vi "Find Turntable Centre.vi"(3 "Mode":T6=enum."Run VI", 5 "Traverse line In":T3={"Start X"=-1250.0, "Start Y"=-250.0, "Start Z"=180.0, "End X"=0.0, "End Y"=0.0, "End Z"=0.0, "No. of pts."=6, "Spacing"=enum."Linear", "Filename"=path "C:/Enflo_Data_Local/2015/EnFlo_Tunnel/Paul_Hayden/Calibrations/Cal_06-2015/Datum_Block_1.xls", "Tunnel Speed"=0.0, "Averaging time (min)"=0.01, "Extra Commands"="", "Carrier_1 Q (l/min)"=nan, "Carrier_2 Q (l/min)"=nan, "Trace Gas Concentration (%)"=nan, "Specific Arguments"="Datum_Image_Calibration.vi  ", "Comments"="", "Row No"=0, "Row Type Selector"=enum."Run VI Named:", "Completion time"="12:51  12-06-2015", "Row Duration (mins)"=0.11291999999999999, "No. of Valid pts."=6, "Meas Setup File"="Trav_Cam_Picture.xls"} {"Carrier_2 Q (l/min)" format="%#.2f"; "Row Duration (mins)" format="%#.1f"; "Row No" min=0; "Trace Gas Concentration (%)" min=0.0 format="%#_4f"; "Carrier_1 Q (l/min)" format="%#.2f"; "Tunnel Speed" format="%#.2f"; "Start X" format="%#.2f"; "Start Y" format="%#.2f"; "Start Z" format="%#.2f"; "End X" format="%#.2f"; "End Y" format="%#.2f"; "End Z" format="%#.2f"; "Averaging time (min)" min=0.0 format="%#.2f"}) -> (0 "Error Message":string, 1 "Status":T2, 2 "Traverse line Out":T3 {"Carrier_2 Q (l/min)" format="%#.2f"; "Row Duration (mins)" format="%#.1f"; "Row No" min=0; "Trace Gas Concentration (%)" min=0.0 format="%#_4f"; "Carrier_1 Q (l/min)" format="%#.2f"; "Tunnel Speed" format="%#.2f"; "Start X" format="%#.2f"; "Start Y" format="%#.2f"; "Start Z" format="%#.2f"; "End X" format="%#.2f"; "End Y" format="%#.2f"; "End Z" format="%#.2f"; "Averaging time (min)" min=0.0 format="%#.2f"})   [LabVIEW 2015]
uses:
  Gen Trav/Traverse_cluster.ctl
  Gen Trav/Spacing.ctl
  Controls/Multi_run_mode.ctl
  Controls/User_Specific_mode.ctl
  Gen Trav/Multi_Run_Status.ctl
  Camera Server/Camera enum/Camera enum.ctl
  Utilities/Image acquisition and processing/Feature detection/Typedefs/Top level controls.ctl
  Utilities/Image acquisition and processing/Feature detection/Typedefs/Theta range.ctl
  Utilities/Image acquisition and processing/Feature detection/Typedefs/Txy range.ctl
  Utilities/Image acquisition and processing/Feature detection/Typedefs/ROI bounds.ctl
  Controls/Setup.ctl
  Controls/Save_Data.ctl
  Globals/Trav_pos_global.vi
  Globals/Constants_global.vi
  Globals/Dynamic_call_global.ph.vi
panel:
  in  "Camera":T1="Travcam"
  out "Local Log File":path
  out "y radius":dbl
  out "x radius":dbl
  out "y centre 2":dbl
  out "x centre 2":dbl
  in  "stop":bool
  out "radius":dbl
  out "y centre":dbl
  out "x centre":dbl
  out "Y":dbl[](array[numeric])
  out "X":dbl[](array[numeric])
  in  "X Offset from Camera":dbl=50.0
  in  "Radius":dbl=500.0
  # "Circle"
  # "Ellipse"
  # "X           Y            Z"
  # "Start"
  # "End"
  # "X           Y            Z"
  # "Start"
  # "End"
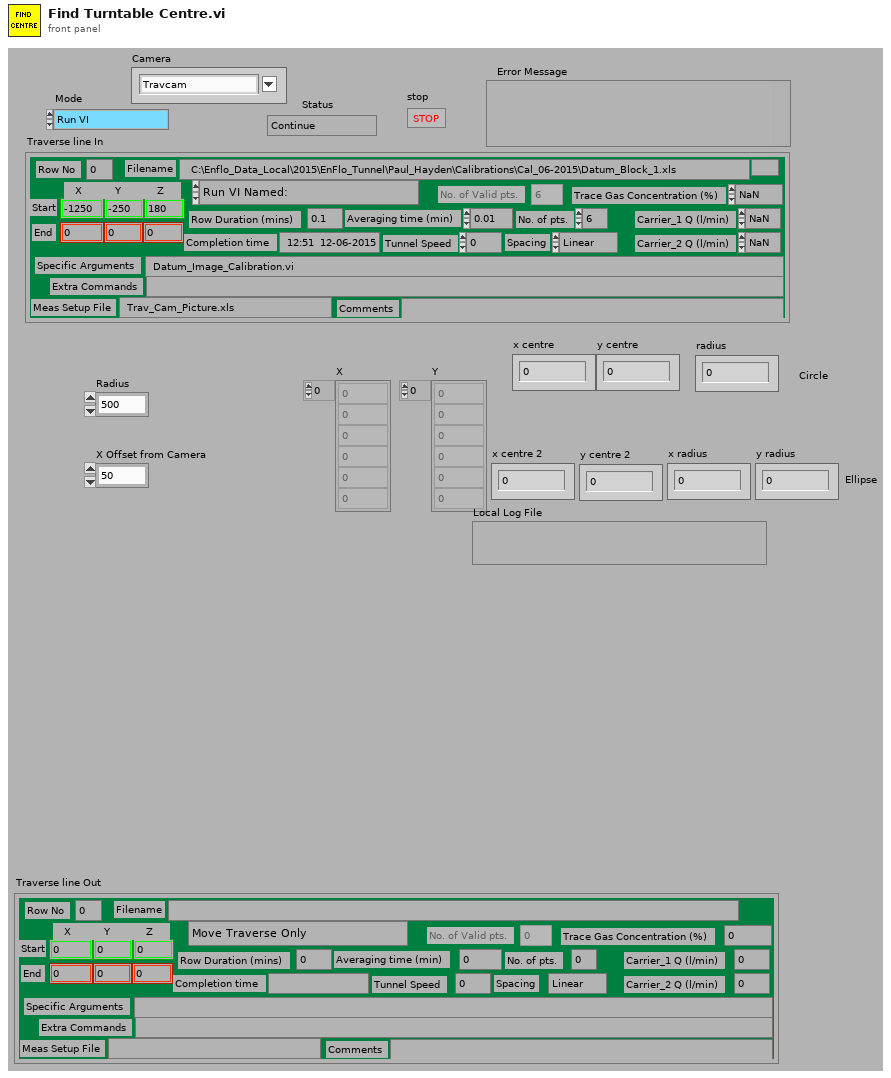
[diagram p1: front panel]
types:
  T1 = typedef "Camera enum.ctl" = string
  T2 = typedef "Multi_Run_Status.ctl" = enum16{"Continue", "Jump to Next Point", "Jump to Next Row", "Jump To Fall Back", "Terminate Run"}
  T3 = typedef "Traverse_cluster.ctl" = cluster{"Start X":sgl, "Start Y":sgl, "Start Z":sgl, "End X":sgl, "End Y":sgl, "End Z":sgl, "No. of pts.":i32, "Spacing":T4, "Filename":path, "Tunnel Speed":dbl, "Averaging time (min)":dbl, "Extra Commands":string, "Carrier_1 Q (l/min)":dbl, "Carrier_2 Q (l/min)":dbl, "Trace Gas Concentration (%)":dbl, "Specific Arguments":string, "Comments":string, "Row No":i32, "Row Type Selector":T5, "Completion time":string, "Row Duration (mins)":dbl, "No. of Valid pts.":i32, "Meas Setup File":string}
  T4 = typedef "Spacing.ctl" = enum16{"Linear", "Log", "Gauss", "Specified", "N/A"}
  T5 = typedef "Multi_run_mode.ctl" = enum16{"Move Traverse Only", "Set Tunnel Speed Only", "Set Source Only", "Set Measurement Conditions", "Single Measurement", "Vertical Profile", "Lateral Profile", "Longitudinal Profile", "Explore Volume", "Multi-Axis Profile", "Auto Calibrate", "Meas Fast FID Bkgnd", "Check Beam Power", "Scanning Valve Measurement", "Run VI Named:", "Set ADAM Ch", "Wait (minutes)", "Send Message", "Synchronize With:", "Fall Back to this Row", "Turn Off Row Repeating", "Blank Row", "Traverse 3D Volume"}
  T6 = typedef "User_Specific_mode.ctl" = enum16{"Check VI only", "Run VI"}
  T7 = typedef "ROI bounds.ctl" = cluster{"Xmax":i32, "Ymax":i32, "Xmin":i32, "Ymin":i32}
  T8 = typedef "Txy range.ctl" = cluster{"Tx max (pix)":i32, "Tx min (pix)":i32, "Ty max (pix)":i32, "Ty min (pix)":i32}
  T9 = typedef "Theta range.ctl" = cluster{"theta max (deg)":dbl, "theta min (deg)":dbl}
  T10 = typedef "Top level controls.ctl" = cluster{"Auto ROI (for rot.)":bool, "Apply scaling":bool, "Apply rotation":bool, "Apply Tx":bool, "Apply Ty":bool, "Keep proc. img":bool}
  T11 = typedef "Save_Data.ctl" = enum16{"Save No Data", "Save Data"}
  T12 = typedef "Setup.ctl" = enum16{"Run Program", "Show Setup", "Save Current Setup", "Setup Front Panel"}
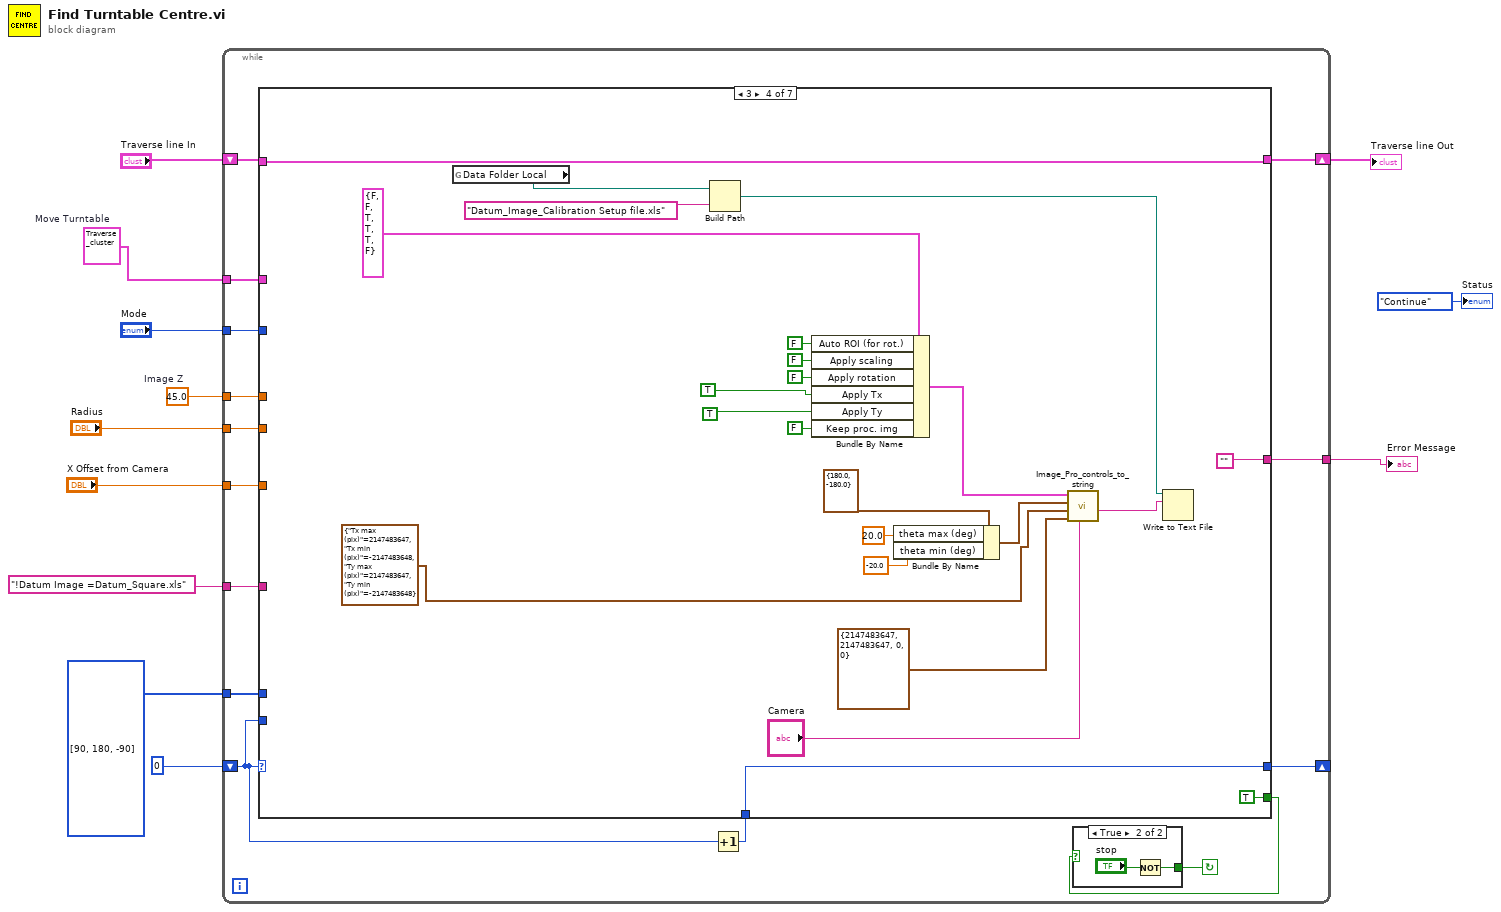
[diagram p0: block diagram]
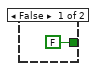
[diagram p2: hidden frame]
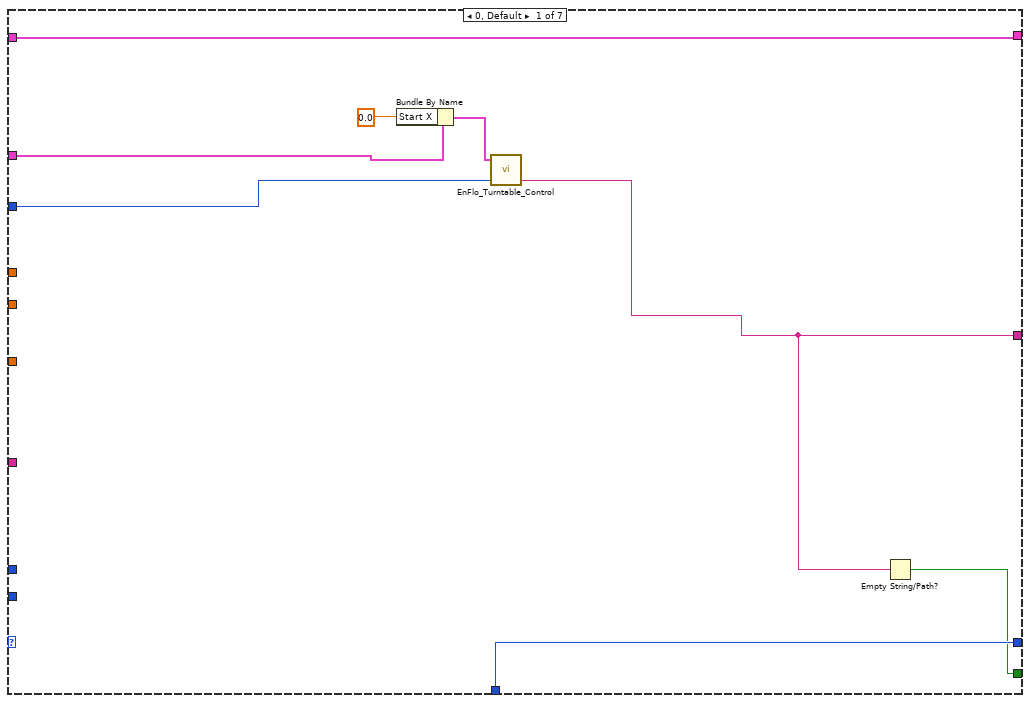
[diagram p3: hidden frame]
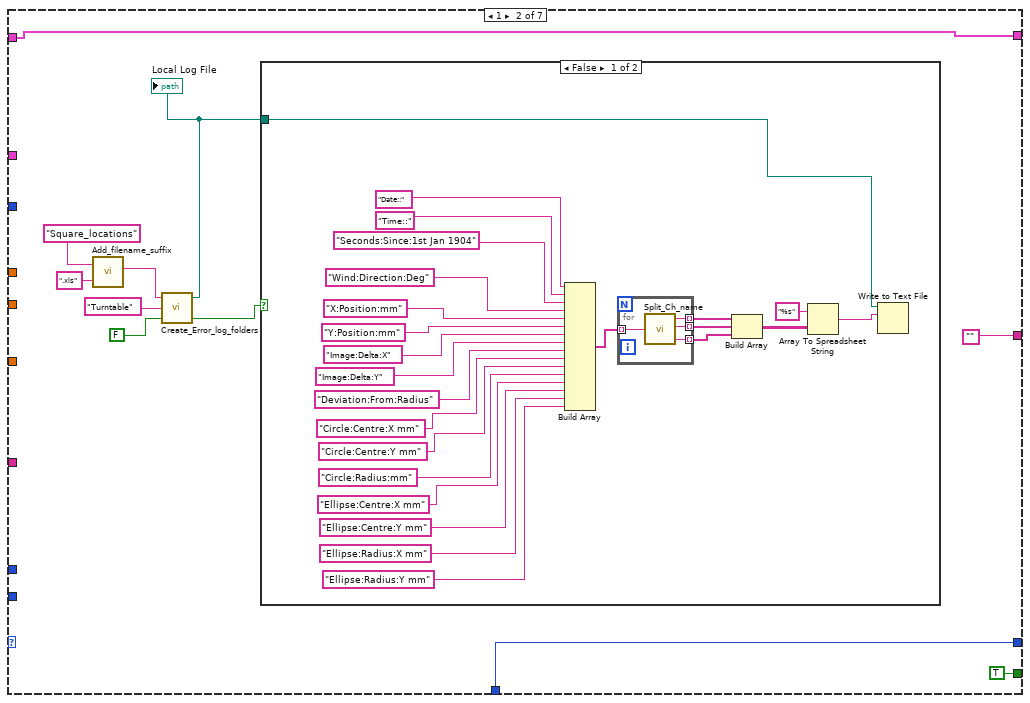
[diagram p4: hidden frame]
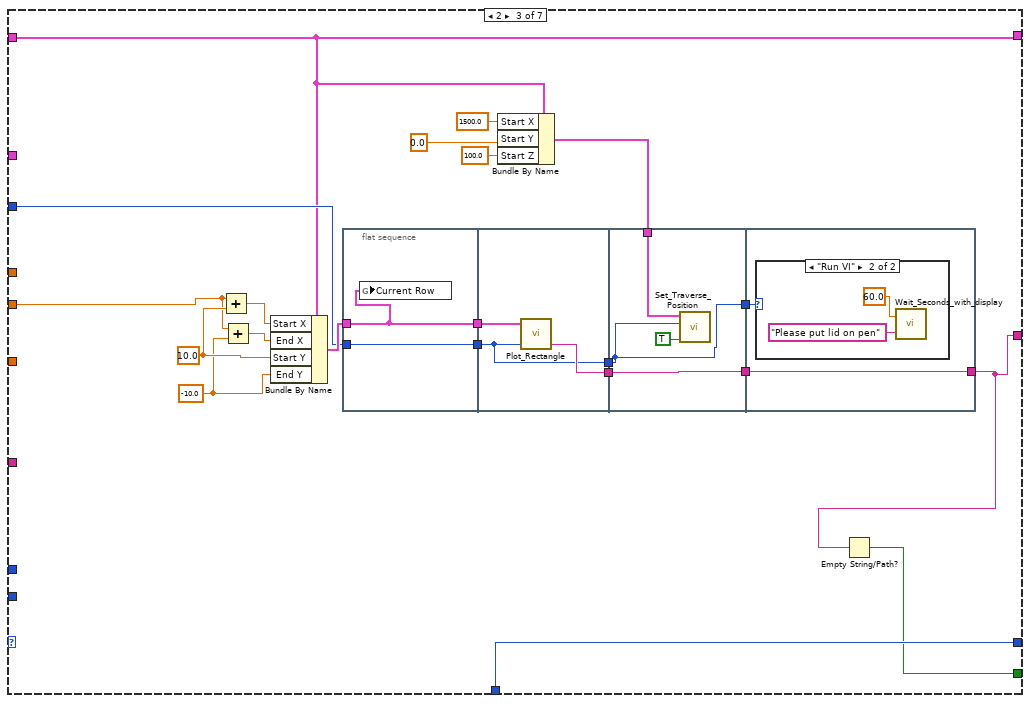
[diagram p6: hidden frame]
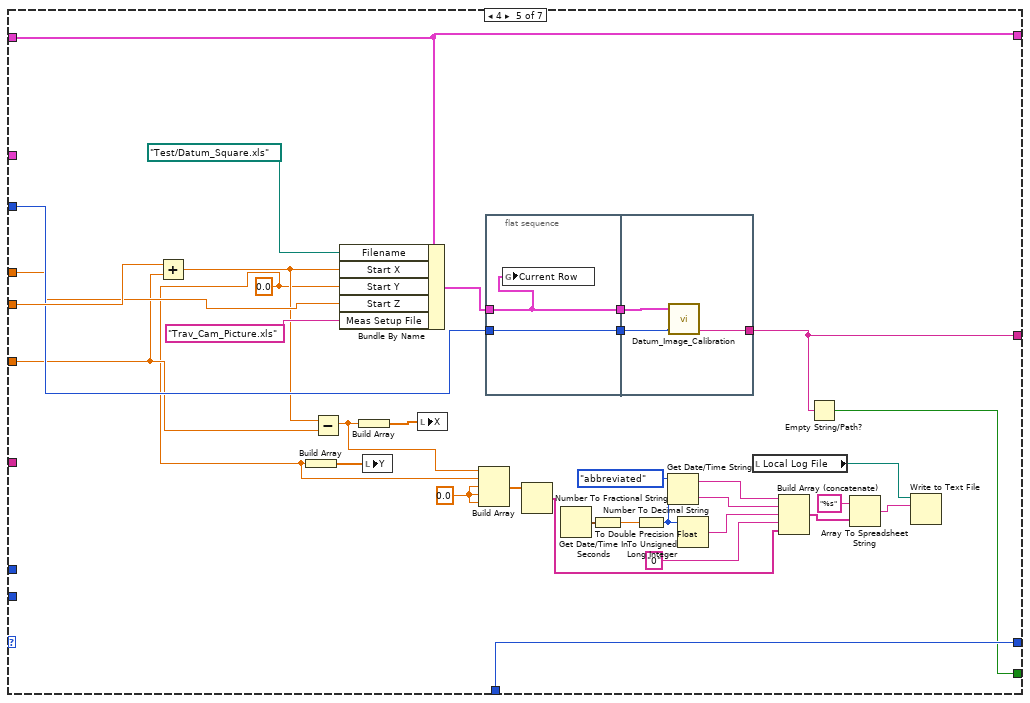
[diagram p8: hidden frame]
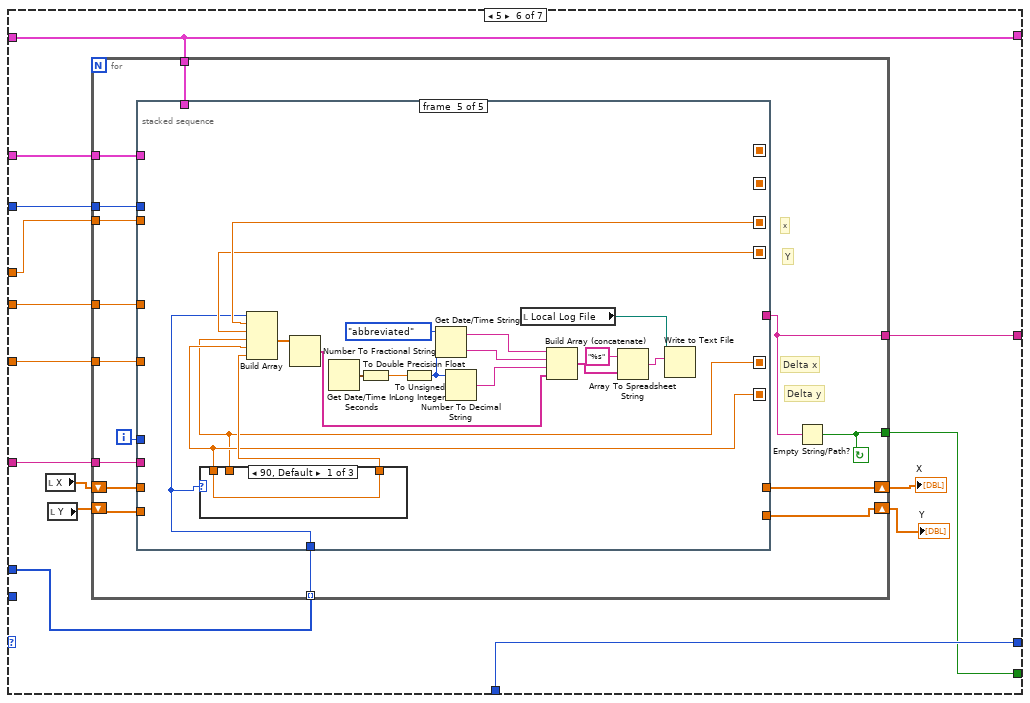
[diagram p9: hidden frame]
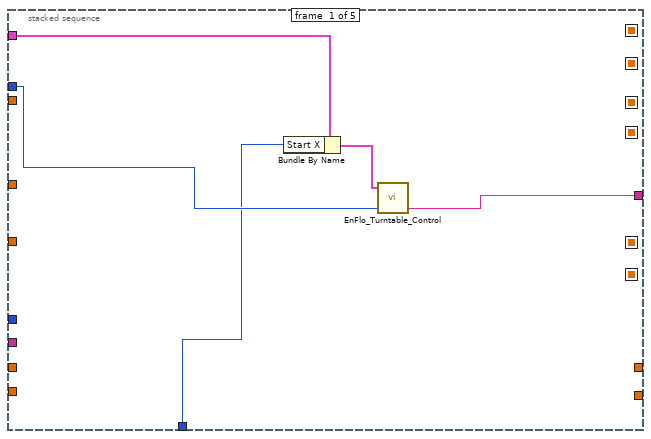
[diagram p10: hidden frame]
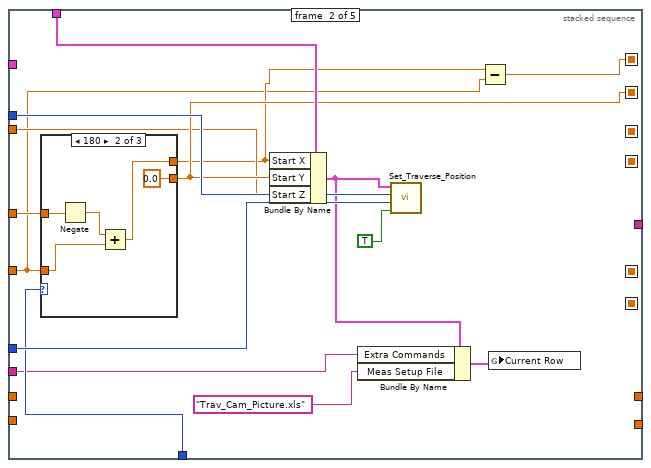
[diagram p11: hidden frame]
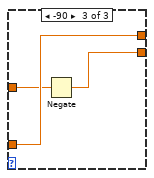
[diagram p13: hidden frame]
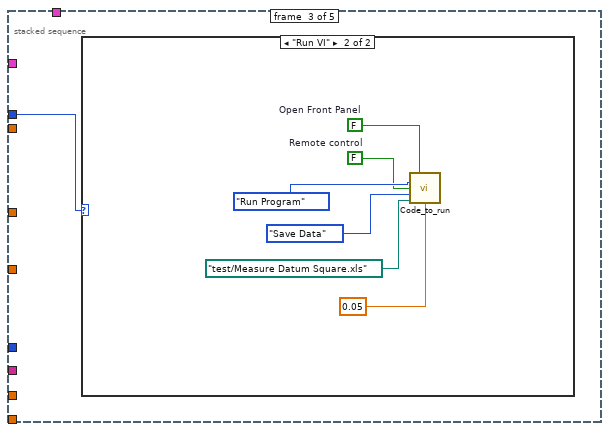
[diagram p14: hidden frame]
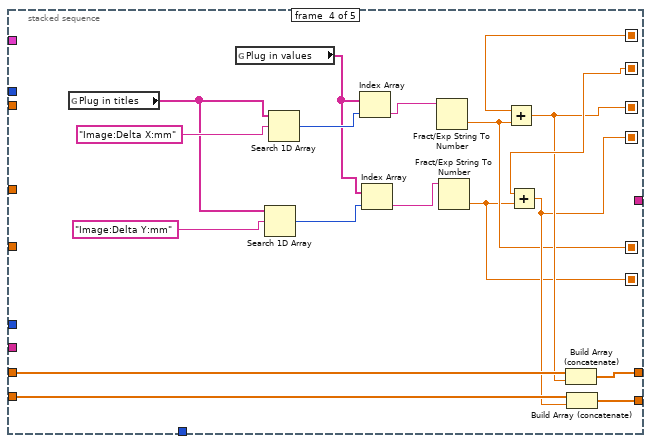
[diagram p16: hidden frame]
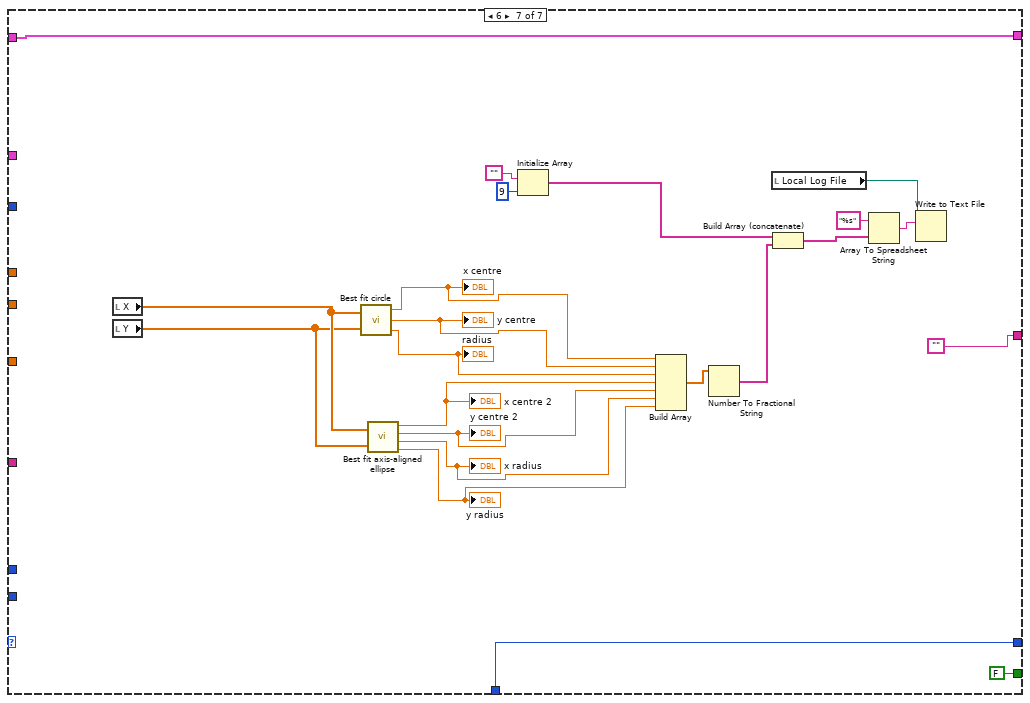
[diagram p19: hidden frame]
diagram:
  w1 = T3 {"Start X"=0.0, "Start Y"=nan, "Start Z"=nan, "End X"=nan, "End Y"=nan, "End Z"=nan, "No. of pts."=0, "Spacing"=enum."N/A", "Filename"=path "  ---------", "Tunnel Speed"=nan, "Averaging time (min)"=nan, "Extra Commands"="!Datum Image = Datum_Turntable.xls", "Carrier_1 Q (l/min)"=nan, "Carrier_2 Q (l/min)"=nan, "Trace Gas Concentration (%)"=nan, "Specific Arguments"="EnFlo_Turntable_Control.vi", "Comments"="", "Row No"=0, "Row Type Selector"=enum."Run VI Named:", "Completion time"="18:36  07-04-2016", "Row Duration (mins)"=0.6666666666666666, "No. of Valid pts."=0, "Meas Setup File"="Trav_Cam_Picture.xls"}  # Move Turntable
  w4 = sgl 45.0  # Image Z
  n1 = while {
    shift-left: 0 -> [w23]
    shift-right: [w27] -> _
    tunnel: "Mode" -> [w26]
    shift-right: [w24] -> w9
    shift-left: "Traverse line In" -> [w25]
    tunnel: "Radius" -> [w21]
    tunnel: "X Offset from Camera" -> [w20]
    tunnel: [w19] -> w6
    tunnel: w4 -> [w18]
    tunnel: i32[] [90, 180, -90] ("appended array") -> [w15]
    tunnel: "!Datum Image =Datum_Square.xls" ("Extra Commands") -> [w14]
    tunnel: w1 -> [w13]
    stop <- w16 continue-if-true
    n2 = Increment(x=w23) -> (x+1=w22:i32)
    n3 = case shown="3" w23 {
      tunnel: [w36 TRUE w95 TRUE w162 w184 FALSE] -> w17
      tunnel: [w38 w41 w97 w134 w166 w187 w298] -> w27
      tunnel: w23 -> [_ _ _ _ _ _ _]
      tunnel: w26 -> [w35 _ w96 _ w158 w186 _]
      tunnel: w25 -> [w37 w42 w86 w133 w167 w181 w299]
      tunnel: [w37 w42 w86 w133 w167 w181 w299] -> w24
      tunnel: w22 -> [w38 w41 w97 w134 w166 w187 w298]
      tunnel: w21 -> [_ _ w89 _ w164 w182 _]
      tunnel: w20 -> [_ _ _ _ w144 w183 _]
      tunnel: [w32 "" w79 "" w157 w185 ""] -> w19
      tunnel: w18 -> [_ _ _ _ w154 w176 _]
      tunnel: w15 -> [_ _ _ _ _ w175 _]
      tunnel: w14 -> [_ _ _ _ _ w174 _]
      tunnel: w13 -> [w31 _ _ _ _ w173 _]
      frame 0, Default {
        n4 = Bundle By Name(cluster=w31, "Start X"=sgl 0.0 ("element")) -> (w34:T3)
        n5 = call "EnFlo_Turntable_Control.vi"("Mode"=w35, "Traverse line In"=w34) -> ("Error Message"=w32:string)  [unwired: 1 in, 2 out]
        n6 = Empty String/Path?(string/path=w32) -> (empty?=w36:bool)
      }
      frame 1 {
        n7 = call "Add_filename_suffix.vi"("Filename"="Square_locations", "Suffix to add"=".xls") -> ("Filename out"=w47:string)  [unwired: 3 out]
        n8 = call "Create_Error_log_folders.vi"("Per Day Log File?"=FALSE, "Log Folder"="Turntable" ("Input Element"), "Log Filename"=w47) -> ("exists?"=w45:bool, "Local Log File"=w43:path)  [unwired: 1 out]
        "Local Log File" <- w43
        n9 = case shown="False" w45 {
          tunnel: w43 -> [w60 _]
          frame False {
            n10 = Build Array("Date::", "Time::", "Seconds:Since:1st Jan 1904", "Wind:Direction:Deg", "X:Position:mm", "Y:Position:mm", "Image:Delta:X", "Image:Delta:Y", "Deviation:From:Radius", "Circle:Centre:X mm", "Circle:Centre:Y mm", "Circle:Radius:mm", "Ellipse:Centre:X mm", "Ellipse:Centre:Y mm", "Ellipse:Radius:X mm", "Ellipse:Radius:Y mm") -> (w69:string[])
            n11 = for {
              tunnel: w69 -> [w77] mode=indexing
              tunnel: [w76] -> w68 mode=indexing
              tunnel: [w75] -> w67 mode=indexing
              tunnel: [w74] -> w66 mode=indexing
              n12 = call "Split_Ch_name.vi"("Ch name"=w77) -> ("Top level"=w76:string, "Middle"=w75:string, "Low level"=w74:string)
            }
            n13 = Build Array(w68, w67, w66) -> (w58:string[][])
            n14 = Array To Spreadsheet String(array=w58, 3:"%s" ("format string")) -> (spreadsheet string=w57:string)  [unwired: 1 out]
            n15 = Write to Text File(file (use dialog)=w60, text=w57) -> ()  [unwired: 2 in, 3 out]
          }
          frame True {
          }
        }
      }
      frame 2 {
        w90 = sgl -10.0 ("End Y")
        w91 = sgl 10.0 ("Start Y")
        n16 = Add(x=w89, y=w91) -> (x+y=w92:dbl)
        n17 = Add(x=w89, y=w90) -> (x+y=w88:dbl)
        n18 = Bundle By Name(cluster=w86, "Start X"=w92, "End X"=w88, "Start Y"=w91, "End Y"=w90) -> (w98:T3)
        n19 = flat-sequence {
          tunnel: w96 -> [w100]
          tunnel: w98 -> [w99]
          tunnel: [w99] -> w94
          tunnel: [w100] -> w93
          tunnel: w94 -> [w103]
          tunnel: w93 -> [w101]
          tunnel: [w102] -> w87
          tunnel: [w101] -> w81
          tunnel: w87 -> [w107]
          tunnel: w82 -> [w106]
          tunnel: w81 -> [w104]
          tunnel: [w107] -> w80
          tunnel: [w104] -> w78
          tunnel: [w109] -> w79
          tunnel: w80 -> [w109]
          tunnel: w78 -> [w108]
          frame #0 {
            n20 = global write "Trav_pos_global.vi" "Current Row"(w99) -> ()
          }
          frame #1 {
            n21 = call "Plot_Rectangle.vi"("Mode"=w101, "Traverse line In"=w103) -> ("Error Message"=w102:string)  [unwired: 1 in, 2 out]
          }
          frame #2 {
            n22 = call "Set_Traverse_Position.vi"("Last Part of Move?"=TRUE, "Simulate/Run"=w104, "Traverse line"=w106) -> ()  [unwired: 3 in, 1 out]
          }
          frame #3 {
            n23 = case shown="\"Run VI\"" w108 {
              frame "Check VI only" {
              }
              frame "Run VI" {
                n24 = call "Wait_Seconds_with_display.vi"("Message"="Please put lid on pen", "Seconds to wait"=60.0) -> ()  [unwired: 1 in, 1 out]
              }
            }
          }
        }
        n25 = Bundle By Name(cluster=w86, "Start X"=sgl 1500.0, "Start Y"=sgl 0.0, "Start Z"=sgl 100.0) -> (w82:T3)
        n26 = Empty String/Path?(string/path=w79) -> (empty?=w95:bool)
      }
      frame 3 {
        n27 = global read "Constants_global.vi" "Data Folder Local"() -> (w131:path)
        n28 = Build Path(base path=w131, name or relative path="Datum_Image_Calibration Setup file.xls") -> (appended path=w115:path)
        n29 = Bundle By Name(cluster=T10 {"Auto ROI (for rot.)"=FALSE, "Apply scaling"=FALSE, "Apply rotation"=TRUE, "Apply Tx"=TRUE, "Apply Ty"=TRUE, "Keep proc. img"=FALSE} ("Controls"), "Auto ROI (for rot.)"=FALSE, "Apply scaling"=FALSE, "Apply rotation"=FALSE, "Apply Tx"=TRUE, "Apply Ty"=TRUE, "Keep proc. img"=FALSE) -> (w123:T10)
        n30 = Bundle By Name(cluster=T9 {"theta max (deg)"=180.0, "theta min (deg)"=-180.0} ("Theta range (deg)"), "theta max (deg)"=20.0, "theta min (deg)"=-20.0) -> (w121:T9)
        n31 = call "Image_Pro_controls_to_string.vi"("Camera"="Camera", "ROI to crop (pixels)"=T7 {"Xmax"=2147483647, "Ymax"=2147483647, "Xmin"=0, "Ymin"=0}, "Txy range (pixels)"=T8 {"Tx max (pix)"=2147483647, "Tx min (pix)"=-2147483648, "Ty max (pix)"=2147483647, "Ty min (pix)"=-2147483648}, "Theta range (deg)"=w121, "Controls"=w123) -> ("Setup String"=w116:string)  [unwired: 6 in]
        n32 = Write to Text File(file (use dialog)=w115, text=w116) -> ()  [unwired: 2 in, 3 out]
      }
      frame 4 {
        w141 = 0.0 ("element")
        w142 = sgl 0.0 ("Start Y")
        n33 = Add(x=w164, y=w144) -> (x+y=w145:dbl)
        n34 = Build Array(w142) -> (w155:sgl[])
        n35 = Subtract(x=w145, y=w144) -> (x-y=w143:dbl)
        n36 = Bundle By Name(cluster=w167, "Filename"=path "Test/Datum_Square.xls", "Start X"=w145, "Start Y"=w142, "Start Z"=w154, "Meas Setup File"="Trav_Cam_Picture.xls") -> (w159:T3)
        n37 = Build Array(w143) -> (w156:dbl[])
        n38 = local write "Y"(w155) -> ()
        n39 = local write "X"(w156) -> ()
        n40 = Build Array(w143, w142, w141, w141, w141) -> (w140:dbl[])
        n41 = flat-sequence {
          tunnel: w158 -> [w169]
          tunnel: w159 -> [w168]
          tunnel: [w168] -> w161
          tunnel: [w169] -> w160
          tunnel: [w170] -> w157
          tunnel: w161 -> [w172]
          tunnel: w160 -> [w171]
          frame #0 {
            n42 = global write "Trav_pos_global.vi" "Current Row"(w168) -> ()
          }
          frame #1 {
            n43 = call "Datum_Image_Calibration.vi"("Mode"=w171, "Traverse line In"=w172) -> ("Error Message"=w170:string)  [unwired: 1 in, 2 out]
          }
        }
        n44 = Number To Fractional String(number=w140) -> (F-format string=w139:string[])  [unwired: 3 in]
        n45 = Get Date/Time In Seconds() -> (seconds since 1Jan1904=w150:timestamp)
        n46 = To Double Precision Float(number=w150) -> (double precision float=w152:dbl)
        n47 = To Unsigned Long Integer(number=w152) -> (unsigned 32bit integer=w151:u32)
        n48 = Get Date/Time String(date format (0)=enum16{"short", "long", "abbreviated"}."abbreviated", seconds (now)=w151) -> (date string=w149:string, time string=w148:string)  [unwired: 1 out]
        n49 = Number To Decimal String(number=w151) -> (decimal integer string=w147:string)  [unwired: 1 out]
        n50 = local read "Local Log File"() -> (w138:path)
        n51 = Build Array (concatenate)(w149, w148, w147, "0", w139) -> (w136:string[])
        n52 = Empty String/Path?(string/path=w157) -> (empty?=w162:bool)
        n53 = Array To Spreadsheet String(array=w136, 3:"%s" ("format string")) -> (spreadsheet string=w135:string)  [unwired: 1 out]
        n54 = Write to Text File(file (use dialog)=w138, text=w135) -> ()  [unwired: 2 in, 3 out]
      }
      frame 5 {
        n55 = local read "X"() -> (w180:dbl[])
        n56 = local read "Y"() -> (w179:dbl[])
        n57 = for {
          tunnel: w186 -> [w202]
          tunnel: [w201] -> w185
          tunnel: [w200] -> w184
          tunnel: w175 -> [w199] mode=indexing
          tunnel: w183 -> [w198]
          tunnel: w182 -> [w197]
          tunnel: w181 -> [w196]
          shift-right: [w192] -> w178
          shift-left: w180 -> [w194]
          shift-right: [w191] -> w177
          shift-left: w179 -> [w193]
          tunnel: w176 -> [w190]
          tunnel: w174 -> [w189]
          tunnel: w173 -> [w188]
          i -> [w195]
          stop <- w200 continue-if-true
          # "Delta y"
          # "Delta x"
          # "Y"
          # "x"
          n58 = stacked-sequence {
            seq-local: [_ w211 _ _ _] -> [_ _ _ w249 _]
            seq-local: [_ w217 _ _ _] -> [_ _ _ w248 _]
            seq-local: [_ _ _ w243 _] -> [_ _ _ _ w263]
            seq-local: [_ _ _ w242 _] -> [_ _ _ _ w262]
            seq-local: [_ _ _ w241 _] -> [_ _ _ _ w258]
            seq-local: [_ _ _ w240 _] -> [_ _ _ _ w259]
            tunnel: w202 -> [w206 w221 w233 _ _]
            tunnel: [w203 _ _ _ _] -> w201
            tunnel: w199 -> [w205 w209 _ _ w261]
            tunnel: w198 -> [_ w210 _ _ _]
            tunnel: w197 -> [_ w218 _ _ _]
            tunnel: w196 -> [_ w222 _ _ _]
            tunnel: w195 -> [_ w219 _ _ _]
            tunnel: w194 -> [_ _ _ w247 _]
            tunnel: w193 -> [_ _ _ w246 _]
            tunnel: [_ _ _ w245 _] -> w192
            tunnel: [_ _ _ w244 _] -> w191
            tunnel: w190 -> [_ w213 _ _ _]
            tunnel: w189 -> [_ w208 _ _ _]
            tunnel: w188 -> [w204 _ _ _ _]
            frame #0 {
              n59 = Bundle By Name(cluster=w204, "Start X"=w205) -> (w207:T3)
              n60 = call "EnFlo_Turntable_Control.vi"("Mode"=w206, "Traverse line In"=w207) -> ("Error Message"=w203:string)  [unwired: 1 in, 2 out]
            }
            frame #1 {
              n61 = case shown="180" w209 {
                tunnel: w210 -> [w224 w226 w232]
                tunnel: [w224 w225 w232] -> w212
                tunnel: w218 -> [w223 w228 w231]
                tunnel: [w223 0.0 ("X position") w230] -> w217
                frame 90, Default {
                }
                frame 180 {
                  n62 = Negate(x=w228) -> (-x=w227:dbl)
                  n63 = Add(x=w227, y=w226) -> (x+y=w225:dbl)
                }
                frame -90 {
                  n64 = Negate(x=w231) -> (-x=w230:dbl)
                }
              }
              n65 = Bundle By Name(cluster=w222, "Start X"=w212, "Start Y"=w217, "Start Z"=w213) -> (w216:T3)
              n66 = Bundle By Name(cluster=w216, "Extra Commands"=w208, "Meas Setup File"="Trav_Cam_Picture.xls" ("Extra Commands")) -> (w215:T3)
              n67 = call "Set_Traverse_Position.vi"("Last Part of Move?"=TRUE, "Currently on Point"=w219, "Simulate/Run"=w221, "Traverse line"=w216) -> ()  [unwired: 2 in, 1 out]
              n68 = Subtract(x=w212, y=w210) -> (x-y=w211:dbl)
              n69 = global write "Trav_pos_global.vi" "Current Row"(w215) -> ()
            }
            frame #2 {
              n70 = case shown="\"Run VI\"" w233 {
                frame "Check VI only" {
                }
                frame "Run VI" {
                  w237 = FALSE  # Open Front Panel
                  w236 = FALSE  # Remote control
                  n71 = call "Code_to_run.vi"("Open Front Panel"=w237, "setup"=Setup."Run Program", "Remote control"=w236, "File"=Save_Data."Save Data", "Results Filename"=path "test/Measure Datum Square.xls", "Averaging time (min)"=0.05) -> ()  [unwired: 5 in, 5 out]
                }
              }
            }
            frame #3 {
              n72 = global read "Dynamic_call_global.ph.vi" "Plug in titles"() -> (w253:string[])
              n73 = global read "Dynamic_call_global.ph.vi" "Plug in values"() -> (w252:string[])
              n74 = Search 1D Array(1D array=w253, element="Image:Delta Y:mm") -> (index of element=w251:i32)  [unwired: 1 in]
              n75 = Search 1D Array(1D array=w253, element="Image:Delta X:mm") -> (index of element=w256:i32)  [unwired: 1 in]
              n76 = Index Array(array=w252, index=w256) -> (element=w257:string)
              n77 = Index Array(array=w252, index=w251) -> (element=w250:string)
              n78 = Fract/Exp String To Number(string=w257) -> (number=w241:dbl)  [unwired: 3 in, 1 out]
              n79 = Fract/Exp String To Number(string=w250) -> (number=w240:dbl)  [unwired: 3 in, 1 out]
              n80 = Add(x=w249, y=w241) -> (x+y=w243:dbl)
              n81 = Add(x=w248, y=w240) -> (x+y=w242:dbl)
              n82 = Build Array (concatenate)(w247, w243) -> (w245:dbl[])
              n83 = Build Array (concatenate)(w246, w242) -> (w244:dbl[])
            }
            frame #4 {
              n84 = case shown="90, Default" w261 {
                tunnel: [w277 w278 w279] -> w260
                tunnel: w259 -> [w277 w278 _]
                tunnel: w258 -> [_ _ w279]
                frame 90, Default {
                }
                frame -90 {
                }
                frame 180 {
                }
              }
              n85 = Build Array(w261, w263, w262, w258, w259, w260) -> (w269:dbl[])
              n86 = Number To Fractional String(number=w269) -> (F-format string=w268:string[])  [unwired: 3 in]
              n87 = Get Date/Time In Seconds() -> (seconds since 1Jan1904=w273:timestamp)
              n88 = To Double Precision Float(number=w273) -> (double precision float=w275:dbl)
              n89 = To Unsigned Long Integer(number=w275) -> (unsigned 32bit integer=w274:u32)
              n90 = Get Date/Time String(date format (0)=enum16{"short", "long", "abbreviated"}."abbreviated", seconds (now)=w274) -> (date string=w272:string, time string=w271:string)  [unwired: 1 out]
              n91 = Number To Decimal String(number=w274) -> (decimal integer string=w270:string)  [unwired: 1 out]
              n92 = local read "Local Log File"() -> (w267:path)
              n93 = Build Array (concatenate)(w272, w271, w270, w268) -> (w265:string[])
              n94 = Array To Spreadsheet String(array=w265, 3:"%s" ("format string")) -> (spreadsheet string=w264:string)  [unwired: 1 out]
              n95 = Write to Text File(file (use dialog)=w267, text=w264) -> ()  [unwired: 2 in, 3 out]
            }
          }
          n96 = Empty String/Path?(string/path=w201) -> (empty?=w200:bool)
        }
        "X" <- w178
        "Y" <- w177
      }
      frame 6 {
        n97 = local read "X"() -> (w297:dbl[])
        n98 = local read "Y"() -> (w296:dbl[])
        n99 = call "Best fit circle.vi"("x array"=w297, "y array"=w296) -> ("x centre"=w288:dbl, "y centre"=w287:dbl, "radius"=w286:dbl)
        "x centre" <- w288
        "y centre" <- w287
        "radius" <- w286
        n100 = call "Best fit axis-aligned ellipse.vi"("x array"=w297, "y array"=w296) -> ("x centre"=w285:dbl, "y centre"=w284:dbl, "x radius"=w283:dbl, "y radius"=w282:dbl)
        "x centre 2" <- w285
        "y centre 2" <- w284
        "x radius" <- w283
        "y radius" <- w282
        n101 = Initialize Array("", 9 ("dimension size")) -> (w280:string[])
        n102 = Build Array(w288, w287, w286, w285, w284, w283, w282) -> (w281:dbl[])
        n103 = Number To Fractional String(number=w281) -> (F-format string=w295:string[])  [unwired: 3 in]
        n104 = local read "Local Log File"() -> (w294:path)
        n105 = Build Array (concatenate)(w280, w295) -> (w292:string[])
        n106 = Array To Spreadsheet String(array=w292, 3:"%s" ("format string")) -> (spreadsheet string=w291:string)  [unwired: 1 out]
        n107 = Write to Text File(file (use dialog)=w294, text=w291) -> ()  [unwired: 2 in, 3 out]
      }
    }
    n108 = case shown="True" w17 {
      tunnel: [FALSE ("stop") w29] -> w16
      frame False {
      }
      frame True {
        n109 = Not(x="stop") -> (.not. x?=w29:bool)
      }
    }
  }
  "Traverse line Out" <- w9
  "Error Message" <- w6
  "Status" <- Multi_Run_Status."Continue" ("Status")
